vi "Init IMAQ.vi"(0 "Custom Device In":T3 format="%.0x", 11 "error in (no error)":errorcluster) -> (4 "Custom Device Out":T3 format="%.0x", 6 "Camera Session":T4, 8 "Acquisition Image":T2, 10 "Image Difference":T1, 15 "error out":errorcluster)   [LabVIEW 2012, in "Image Difference Custom Device.lvlib"]
uses:
  Image Difference Custom Device.lvlib
  <vilib>/userdefined/High Color/IMAQdx.ctl
  <vilib>/vision/Image Controls.llb/IMAQ Image.ctl
  <vilib>/NI Veristand/Custom Device API/Custom Device Item Ref.ctl
  TypeDefs/Image Difference Info.ctl
  Image Difference Global.vi
  <vilib>/NI Veristand/Custom Device API/Get Item Property (Variant).vi
  <vilib>/NI Veristand/Custom Device API/Get Item Property (String).vi
  <vilib>/vision/driver/NI_Vision_Acquisition_Software.lvlib
  <resource>/objmgr/imaqdx.rc
  <vilib>/NI Veristand/Custom Device API/Custom Device API.lvlib
  <vilib>/NI Veristand/Custom Device API/Get Item Property (Dependent File).vi
  <vilib>/vision/NI_Vision_Development_Module.lvlib
panel:
  in  "Trigger Parameters (from NIVS)":T5={"Trigger Mode"=6, "Timeout (ms)"=1000, "Trigger Activation"=1} {"Trigger Activation" items=["LevelLow", "LevelHigh"]; "Trigger Mode" items=["Mode0"=0, "Off"=6]}
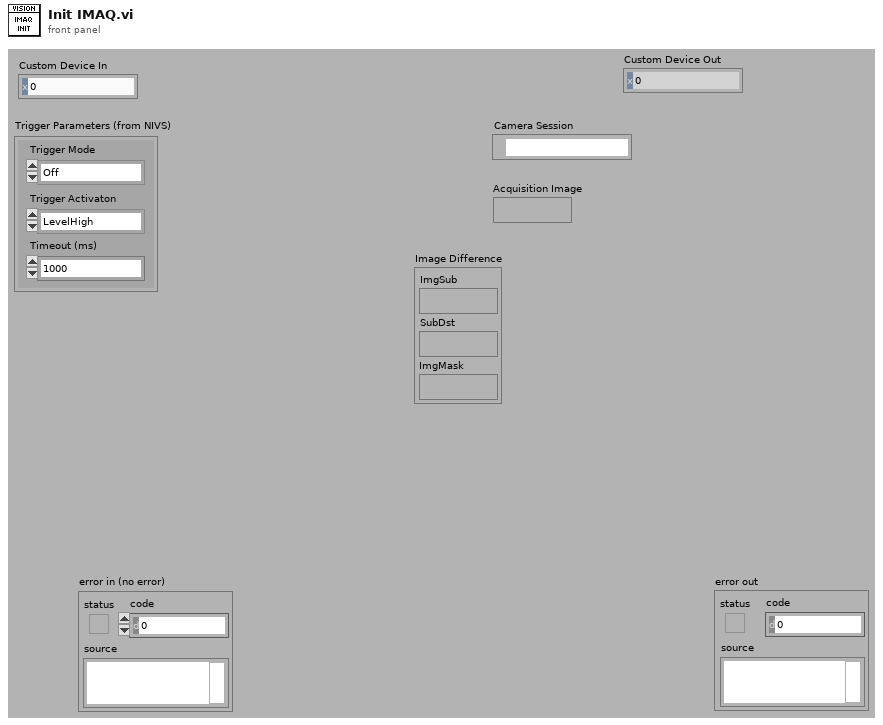
[diagram p1: front panel]
types:
  T1 = typedef "Image Difference Custom Device.lvlib/Image Difference Info.ctl" = cluster{"ImgSub":T2, "SubDst":T2, "ImgMask":T2}
  T2 = typedef "IMAQ Image.ctl" = refnum<image>
  T3 = typedef "Custom Device API.lvlib/Custom Device Item Ref.ctl" = u64
  T4 = typedef "IMAQdx.ctl" = refnum<k21>
  T5 = cluster{"Trigger Mode":u32, "Timeout (ms)":u32, "Trigger Activation":u32}
  T6 = cluster{"Global Rectangle":i32[], "Contours":cluster{"Contour Type":u32, "ROI Type":u32, "Points":i32[]}[]}
  T7 = typedef "Custom Device API.lvlib/Dependent File Optional Info.ctl" = cluster{"Version":string, "RTDestination":path, "ForceDownload":bool, "SupportedTarget":string, "MD5":string}
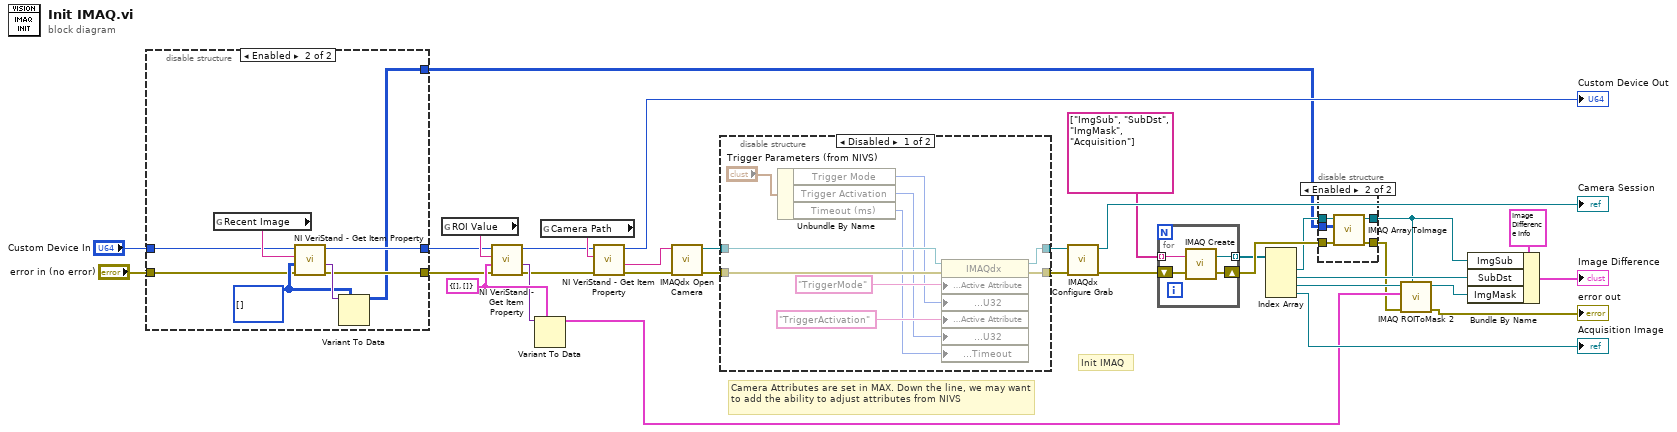
[diagram p0: block diagram]
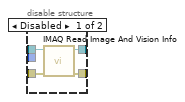
[diagram p2: hidden frame]
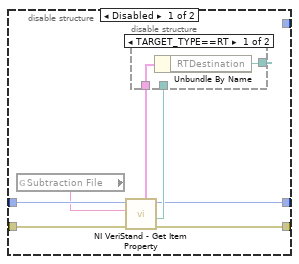
[diagram p3: hidden frame]
diagram:
  w14 = T6 {"Global Rectangle"=[], "Contours"=[]} ("ROI")
  # "Camera Attributes are set in MAX. Down the line, we may want to add the ability to adjust attributes from NIVS"
  # "Init IMAQ"
  n1 = disable-structure shown="Enabled" {
    disable-tunnel: "Custom Device In" -> [w41 w48]
    disable-tunnel: "error in (no error)" -> [w40 w49]
    disable-tunnel: [w36 w47] -> w10
    disable-tunnel: [w35 w46] -> w11
    disable-tunnel: [_ w45] -> w15
    frame Disabled {
      n2 = global read "Image Difference Global.vi" "Subtraction File"() -> (w39:string)
      n3 = call-poly <vilib>:"NI VeriStand - Get Item Property.vi"("error in (no error)"=w40, "Property Name"=w39, "Item Ref in"=w41) -> ("error out"=w35:errorcluster, "Path"=w37:path, "Item Ref out"=w36:T3, "OptionalInfo"=w38:T7)  [unwired: 4 in, 1 out]
      n4 = disable-structure shown="TARGET_TYPE==RT" {
        disable-tunnel: w38 -> [w43 _]
        disable-tunnel: [w42 w44] -> _
        disable-tunnel: w37 -> [_ w44]
        frame condition #0 {
          n5 = Unbundle By Name(w43) -> ("RTDestination"=w42:path)
        }
        frame condition #1 (active) {
        }
      }
    }
    frame Enabled {
      w51 = u8[][] []
      n6 = global read "Image Difference Global.vi" "Recent Image"() -> (w50:string)
      n7 = call-poly <vilib>:"NI VeriStand - Get Item Property.vi"("error in (no error)"=w49, "Default Value"=w51, "Property Name"=w50, "Item Ref in"=w48) -> ("error out"=w46:errorcluster, "Value"=w52:variant, "Item Ref out"=w47:T3)  [unwired: 4 in, 1 out]
      n8 = Variant To Data(type=w51, Variant=w52) -> (data=w45:u8[][])  [unwired: 1 in, 1 out]
    }
  }
  n9 = global read "Image Difference Global.vi" "ROI Value"() -> (w12:string)
  n10 = call-poly <vilib>:"NI VeriStand - Get Item Property.vi"("error in (no error)"=w11, "Default Value"=w14, "Property Name"=w12, "Item Ref in"=w10) -> ("error out"=w9:errorcluster, "Value"=w13:variant, "Item Ref out"=w8:T3)  [unwired: 4 in, 1 out]
  n11 = Variant To Data(type=w14, Variant=w13) -> (data=w5:T6)  [unwired: 1 in, 1 out]
  n12 = global read "Image Difference Global.vi" "Camera Path"() -> (w25:string)
  n13 = call-poly <vilib>:"NI VeriStand - Get Item Property.vi"("error in (no error)"=w9, "Property Name"=w25, "Item Ref in"=w8) -> ("error out"=w24:errorcluster, "Value"=w23:string, "Item Ref out"=→"Custom Device Out":T3)  [unwired: 5 in, 1 out]
  n14 = call <vilib>:"IMAQdx Open Camera.vi"("error in"=w24, "Session In"=w23) -> ("error out"=w28:errorcluster, "Session Out"=w22:T4)  [unwired: 1 in, 7 out]
  n15 = disable-structure shown="Disabled" {
    disable-tunnel: w28 -> [w59 w64]
    disable-tunnel: w22 -> [w58 w63]
    disable-tunnel: [w57 w64] -> w27
    disable-tunnel: [w56 w63] -> w26
    frame Disabled {
      n16 = Unbundle By Name("Trigger Parameters (from NIVS)") -> ("Trigger Mode"=w55:u32, "Trigger Activation"=w54:u32, "Timeout (ms)"=w53:u32)
      n17 = property class="IMAQdx"(reference=w58, error in=w59, "Camera Attributes:Active Attribute"="TriggerMode" ("ActiveAttribute"), "Camera Attributes:Value:U32"=w55, "Camera Attributes:Active Attribute"="TriggerActivation" ("ActiveAttribute"), "Camera Attributes:Value:U32"=w54, "Acquisition Attributes:Timeout"=w53) -> (reference out=w56:T4, error out=w57:errorcluster)
    }
    frame Enabled {
    }
  }
  n18 = call <vilib>:"IMAQdx Configure Grab.vi"("error in"=w27, "Session In"=w26) -> ("error out"=w17:errorcluster, "Session Out"=→"Camera Session":T4)  [unwired: 8 out]
  n19 = for {
    tunnel: string[] ["ImgSub", "SubDst", "ImgMask", "Acquisition"] -> [w68] mode=indexing
    tunnel: [w66] -> w31 mode=indexing
    shift-right: [w65] -> w33
    shift-left: w17 -> [w67]
    n20 = call "IMAQ Create"("Image Name"=w68, "error in (no error)"=w67) -> ("New Image"=w66:T2, "error out"=w65:errorcluster)  [unwired: 2 in, 1 out]
  }
  n21 = Index Array(array=w31) -> (element #1=w32:T2, element #2=w30:T2, element #3=w6:T2, element #4=→"Acquisition Image":T2)  [unwired: 4 in]
  n22 = disable-structure shown="Enabled" {
    disable-tunnel: [w72 w76] -> w1
    disable-tunnel: [w71 w75] -> w4
    disable-tunnel: w33 -> [w70 w74]
    disable-tunnel: w32 -> [w69 w77]
    disable-tunnel: w15 -> [_ w73]
    frame Disabled {
      n23 = call "IMAQ Read Image And Vision Info"("error in (no error)"=w70, "Image"=w69) -> ("error out"=w71:errorcluster, "Image Out"=w72:T2)  [unwired: 7 in, 1 out]
    }
    frame Enabled {
      n24 = call "IMAQ ArrayToImage"("error in (no error)"=w74, "Image Pixels (U8)"=w73, "Image"=w77) -> ("error out"=w75:errorcluster, "Image Out"=w76:T2)  [unwired: 7 in]
    }
  }
  n25 = call "IMAQ ROIToMask 2"("Image Model"=w1, "error in (no error)"=w4, "ROI Descriptor"=w5, "Image"=w6) -> ("error out"=→"error out":errorcluster, "Image Out"=w3:T2)  [unwired: 5 in, 1 out]
  n26 = Bundle By Name(cluster=T1 {"ImgSub"=refnum, "SubDst"=refnum, "ImgMask"=refnum} ("Threshold and Image Subtraction"), "ImgSub"=w1, "SubDst"=w30, "ImgMask"=w3) -> (→"Image Difference":T1)
